vi "data_selector.vi"(10 "数据显示配置":T1, 11 "数组":waveform(dbl)[](array[waveform])) -> (1 "波形输出UI 4":T5, 2 "波形输出UI 3":T5, 3 "波形输出UI 2":T5, 4 "波形输出UI 5":T5, 5 "波形输出UI 1":T5, 6 "波形输出UI 6":T5)   [LabVIEW 2018, in "UI.lvlib"]
uses:
  UI.lvlib
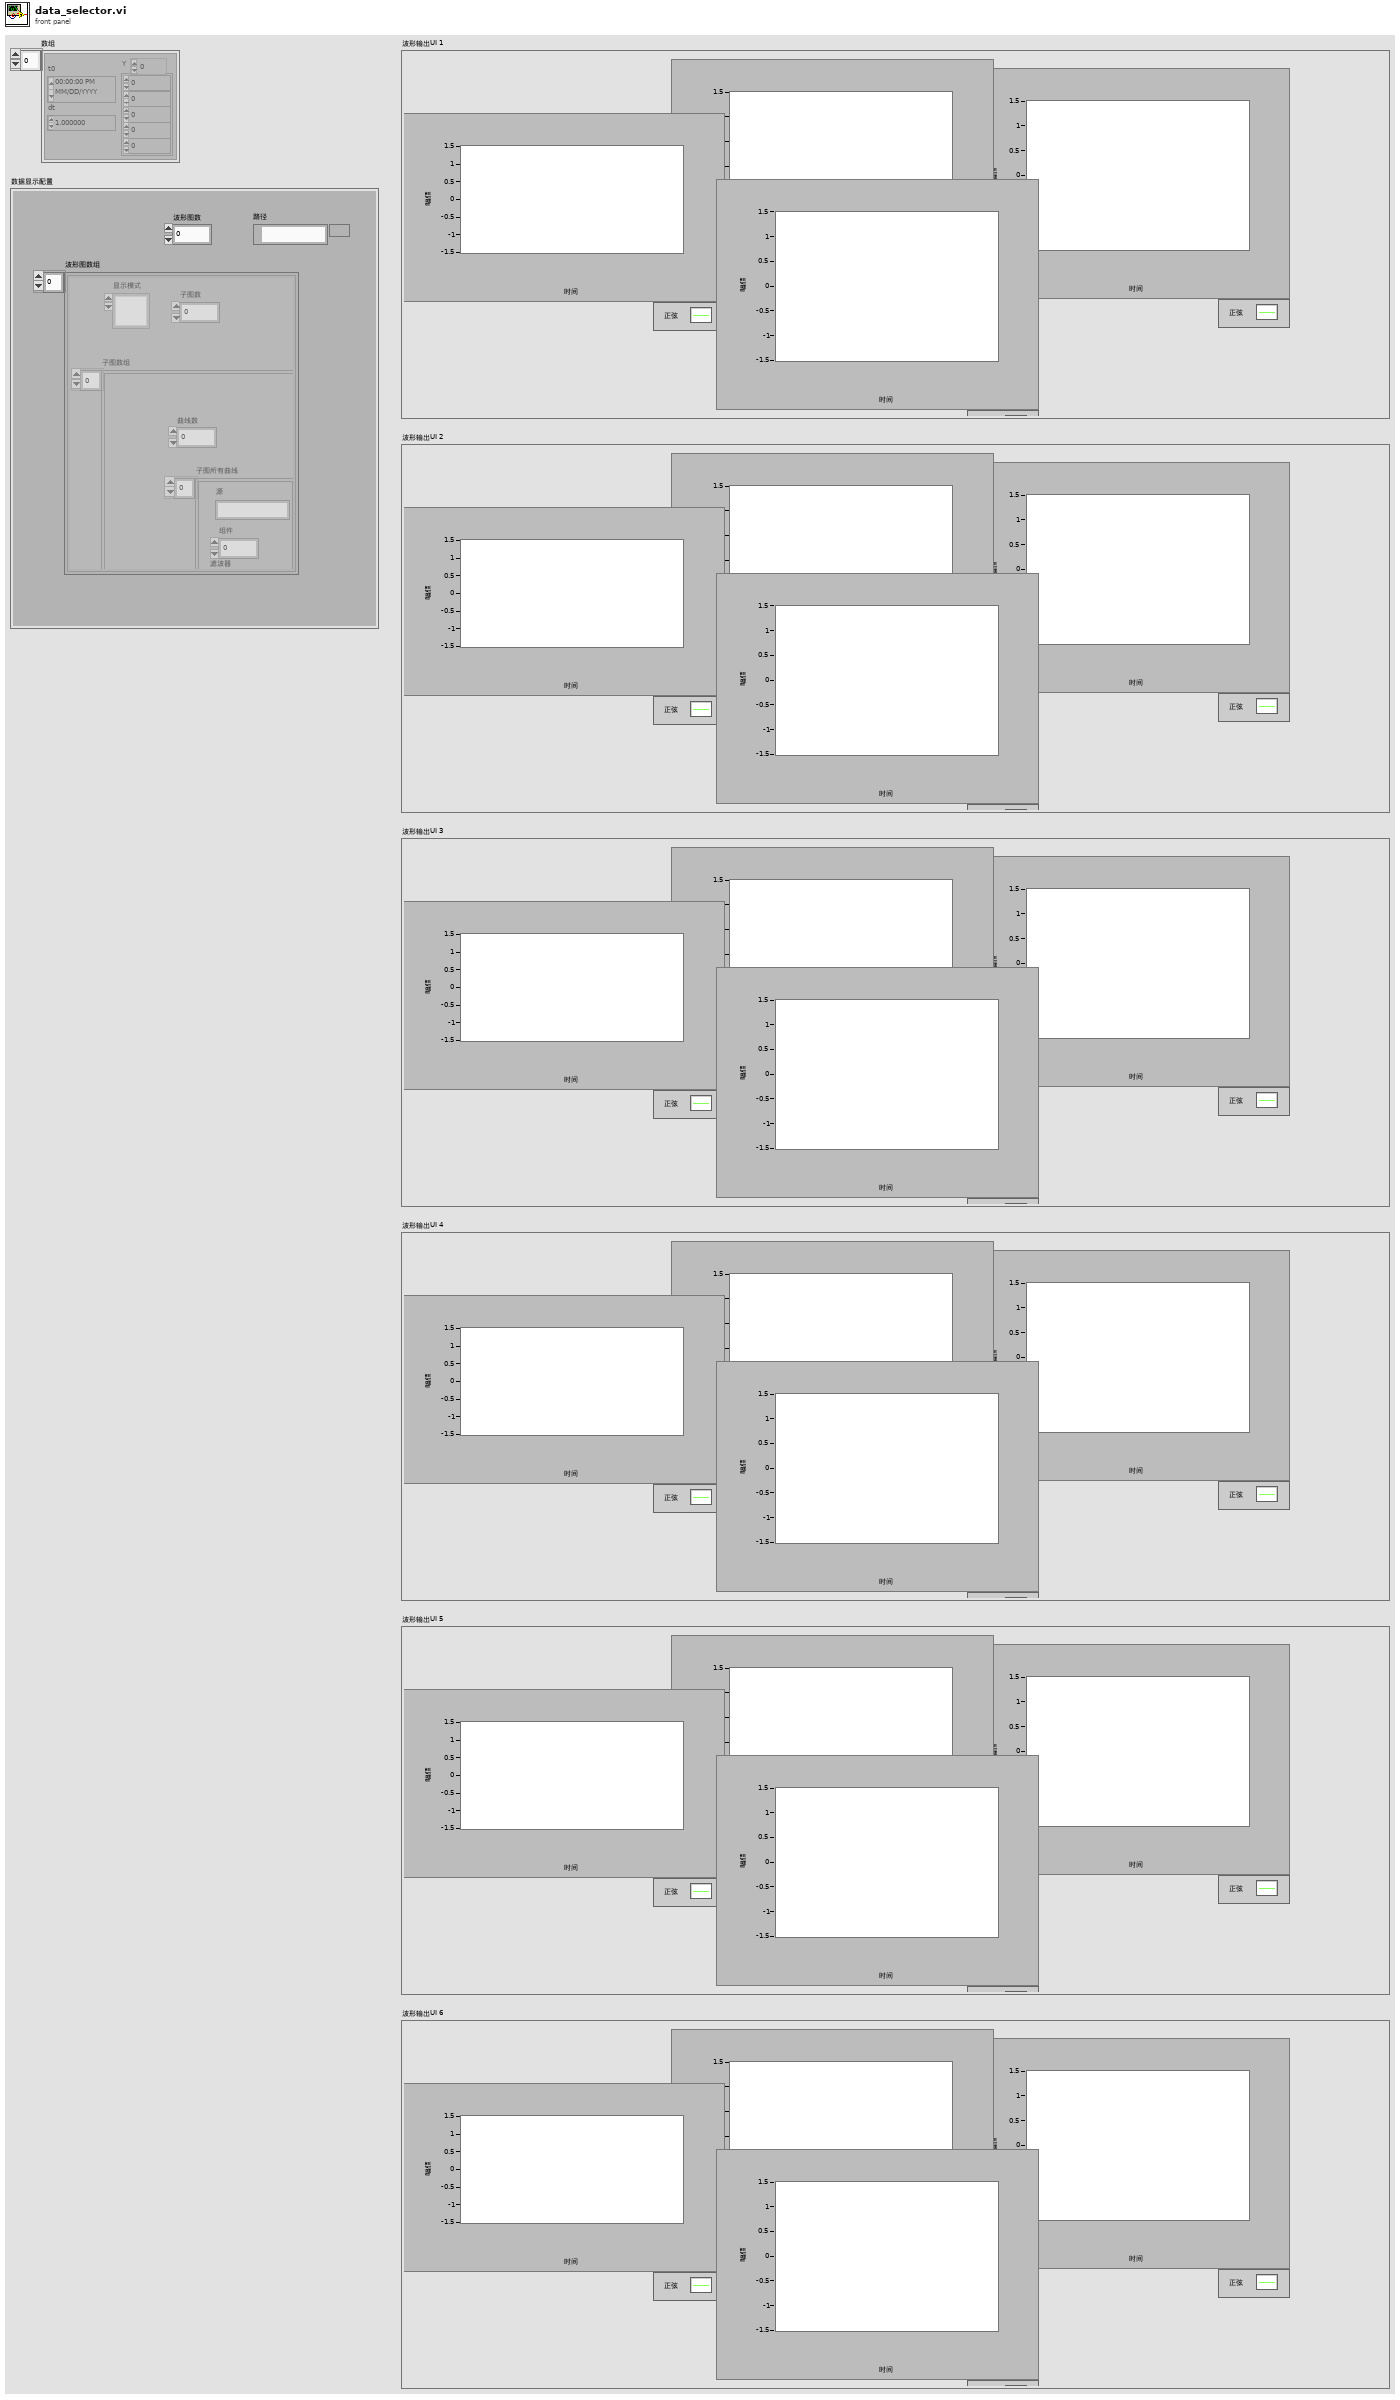
[diagram p1: front panel]
types:
  T1 = typedef "波形图簇.ctl" = cluster{"波形图数":u32, "波形图数组":T2[], "路径":path}
  T2 = typedef "波形图.ctl" = cluster{"显示模式":u16, "子图数":u32, "子图数组":T3[]}
  T3 = typedef "子图.ctl" = cluster{"子图所有曲线":T4[], "曲线数":u32}
  T4 = typedef "曲线簇.ctl" = cluster{"源":string, "组件":u32, "滤波器":u32}
  T5 = typedef "控件 13.ctl" = cluster{"数据 1":waveform(dbl)[], "数据 2":waveform(dbl)[], "数据 3":waveform(dbl)[], "数据 4":waveform(dbl)[]}
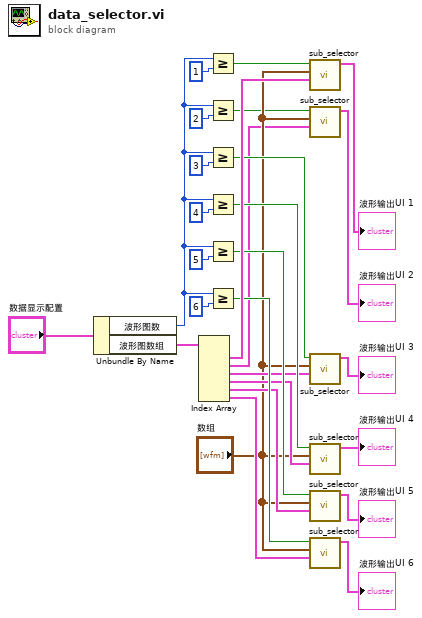
[diagram p0: block diagram]
diagram:
  n1 = Unbundle By Name("数据显示配置") -> ("波形图数"=w20:u32, "波形图数组"=w26:T2[])
  n2 = Index Array(array=w26) -> (element #1=w18:T2, element #2=w2:T2, element #3=w6:T2, element #4=w9:T2, element #5=w12:T2, element #6=w13:T2)  [unwired: 6 in]
  n3 = Greater Or Equal?(x=w20, y=1) -> (x >= y?=w19:bool)
  n4 = Greater Or Equal?(x=w20, y=2) -> (x >= y?=w1:bool)
  n5 = Greater Or Equal?(x=w20, y=3) -> (x >= y?=w5:bool)
  n6 = Greater Or Equal?(x=w20, y=4) -> (x >= y?=w8:bool)
  n7 = Greater Or Equal?(x=w20, y=5) -> (x >= y?=w11:bool)
  n8 = Greater Or Equal?(x=w20, y=6) -> (x >= y?=w14:bool)
  n9 = call "sub_selector.vi"("波形"=w18, "数组"="数组", "布尔"=w19) -> ("波形输出UI 7"=→"波形输出UI 1":T5)  [unwired: 8 in]
  n10 = call "sub_selector.vi"("波形"=w2, "数组"="数组", "布尔"=w1) -> ("波形输出UI 7"=→"波形输出UI 2":T5)  [unwired: 8 in]
  n11 = call "sub_selector.vi"("波形"=w6, "数组"="数组", "布尔"=w5) -> ("波形输出UI 7"=→"波形输出UI 3":T5)  [unwired: 8 in]
  n12 = call "sub_selector.vi"("波形"=w9, "数组"="数组", "布尔"=w8) -> ("波形输出UI 7"=→"波形输出UI 4":T5)  [unwired: 8 in]
  n13 = call "sub_selector.vi"("波形"=w12, "数组"="数组", "布尔"=w11) -> ("波形输出UI 7"=→"波形输出UI 5":T5)  [unwired: 8 in]
  n14 = call "sub_selector.vi"("波形"=w13, "数组"="数组", "布尔"=w14) -> ("波形输出UI 7"=→"波形输出UI 6":T5)  [unwired: 8 in]
